vi "Get EST Tunnel and Diagram Ref.vi"(8 "error in (no error)":errorcluster, 10 "FlatSeq Refnum":refnum<vi>, 11 "Digital High Speed Loop in":refnum<class "Digital High Speed Loop.lvclass">) -> (0 "error out":errorcluster, 3 "Digital High Speed Loop out":refnum<class "Digital High Speed Loop.lvclass">)   [LabVIEW 2015, in "Digital High Speed Loop.lvclass"]
uses:
  Digital High Speed Loop.lvclass
  Structures/Structures.lvclass/Structures.ctl
  Structures/Write Structure.vi
  Module Loop/Write EST Tunnel.vi
  Structures/Write Diagram.vi
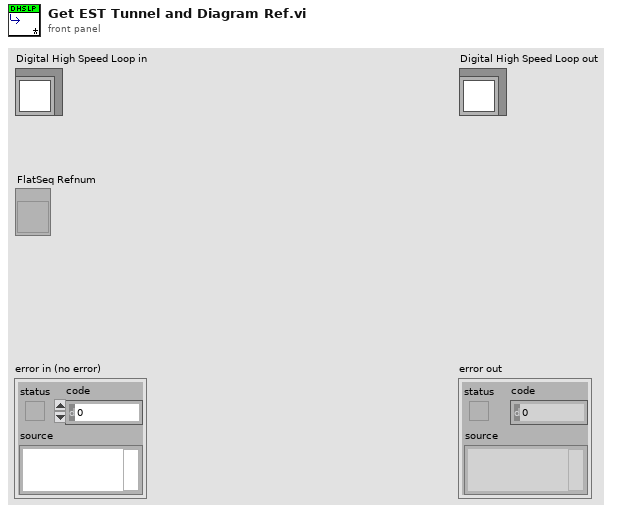
[diagram p1: front panel]
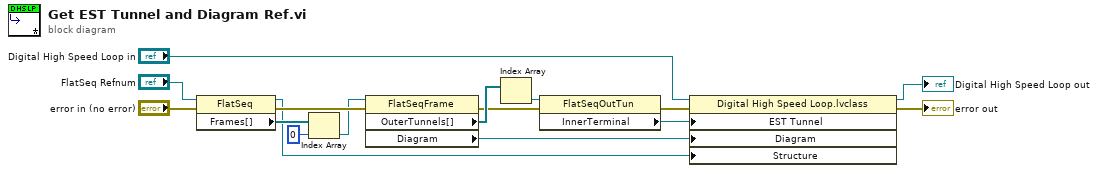
[diagram p0: block diagram]
diagram:
  n1 = property class="FlatSeq"(reference="FlatSeq Refnum", error in="error in (no error)") -> (reference out=w1:refnum<vi>, error out=w14:errorcluster, "Frames[]"=w16:refnum<vi>[])
  n2 = Index Array(array=w16, index=0) -> (element=w2:refnum<vi>)
  n3 = property class="FlatSeqFrame"(reference=w2, error in=w14) -> (error out=w11:errorcluster, "OuterTunnels[]"=w13:refnum<vi>[], "Diagram"=w10:refnum<vi>)  [unwired: 1 out]
  n4 = Index Array(array=w13) -> (element=w12:refnum<vi>)  [unwired: 1 in]
  n5 = property class="FlatSeqOutTun"(reference=w12, error in=w11) -> (error out=w8:errorcluster, "InnerTerminal"=w9:refnum<vi>)  [unwired: 1 out]
  n6 = property class="Digital High Speed Loop.lvclass"(reference="Digital High Speed Loop in", error in=w8, "EST Tunnel"=w9, "Diagram"=w10, "Structure"=w1) -> (reference out=→"Digital High Speed Loop out":refnum<class "Digital High Speed Loop.lvclass">, error out=→"error out":errorcluster)
